vi "FGV_CAN_LOG.vi"(8 "errin":errorcluster, 9 "CMD":T1, 11 "ChaineIn":string) -> (0 "errout":errorcluster, 3 "Chaîne":string)   [LabVIEW 2020]
uses:
  FGV.ctl
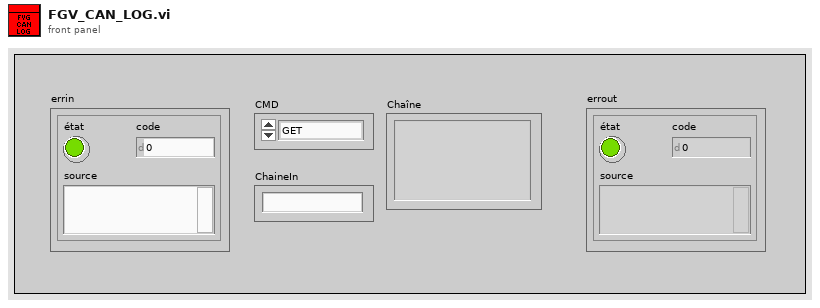
[diagram p1: front panel]
types:
  T1 = typedef "FGV.ctl" = enum16{"GET", "SET", "RAZ"}
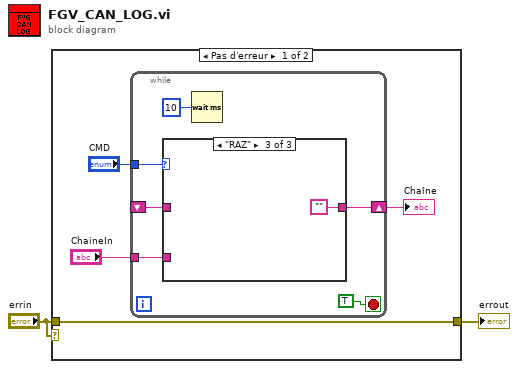
[diagram p0: block diagram]
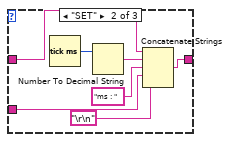
[diagram p3: hidden frame]
diagram:
  n1 = case shown="Pas d'erreur" "errin" {
    tunnel: [w3 w22] -> w2
    tunnel: "errin" -> [w3 w22]
    frame No Error {
      n2 = while {
        tunnel: "CMD" -> [w12]
        shift-right: [w9] -> w5
        shift-left: _ -> [w8]
        tunnel: "ChaineIn" -> [w7]
        stop <- TRUE stop-if-true
        n3 = case shown="\"RAZ\"" w12 {
          tunnel: [w13 w20 ""] -> w9
          tunnel: w8 -> [w13 w15 _]
          tunnel: w7 -> [_ w16 _]
          frame "GET", Default {
          }
          frame "SET" {
            n4 = Tick Count (ms)() -> (millisecond timer value=w19:u32)
            n5 = Number To Decimal String(number=w19) -> (decimal integer string=w18:string)  [unwired: 1 in]
            n6 = Concatenate Strings(w15, w18, "ms : " ("chaîne"), w16, "\r\n") -> (w20:string)
          }
          frame "RAZ" {
          }
        }
        n7 = Wait (ms)(milliseconds to wait=u32 10 ("attente (ms)")) -> ()  [unwired: 1 out]
      }
      "Chaîne" <- w5
    }
    frame Error {
    }
  }
  "errout" <- w2
